vi "Read Repo_Name.vi"(8 "error in (no error)":errorcluster, 11 "VIP Publish in":refnum<class "VIP Publish.lvclass">) -> (0 "error out":errorcluster, 2 "Repo_Name":string, 3 "VIP Publish out":refnum<class "VIP Publish.lvclass">)   [LabVIEW 2014, in "VIP Publish.lvclass"]
uses:
  VIP Publish.lvclass
  VIP Publish.lvclass/VIP Publish.ctl
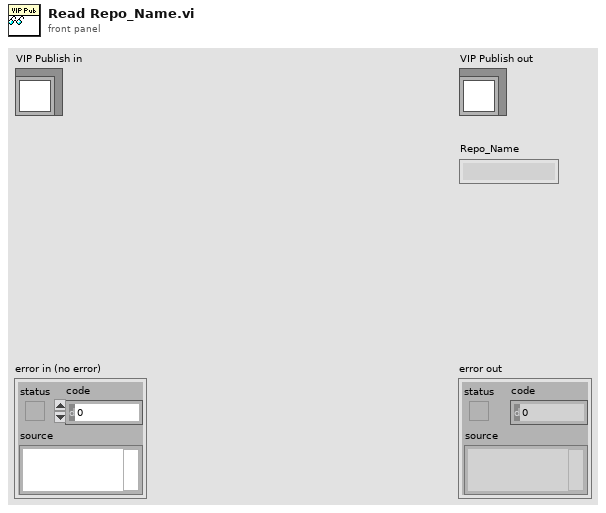
[diagram p1: front panel]
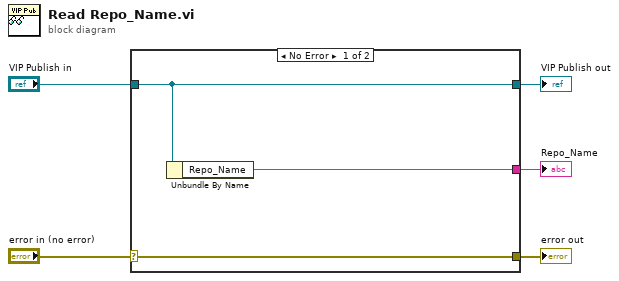
[diagram p0: block diagram]
diagram:
  n1 = case shown="No Error" "error in (no error)" {
    selector: "error in (no error)" -> [w8 w9]
    tunnel: [w8 w9] -> w4
    tunnel: [w7 w10] -> w2
    tunnel: "VIP Publish in" -> [w7 w10]
    tunnel: [w6 _] -> w1
    frame No Error {
      n2 = Unbundle By Name(w7) -> ("Repo_Name"=w6:string)
    }
    frame Error {
    }
  }
  "error out" <- w4
  "VIP Publish out" <- w2
  "Repo_Name" <- w1
